vi "merFISH_resume.vi"(7 "Queue cluster":T2, 8 "Input data cluster":T1, 10 "error in":errorcluster, 11 "merFISH path":path=path "E:/") -> (1 "refnum log file":refnum<file>, 2 "Ramp":dbl[](array[numeric]), 3 "Total # z steps":i32, 4 "Ready":bool, 5 "Total # frames":i32, 6 "error out":errorcluster)   [LabVIEW 2015]
uses:
  CONTROLS/Q_PUMP_element.ctl
  CONTROLS/Q_VALVE_element.ctl
  CONTROLS/Q_DAQ_element.ctl
  CONTROLS/Q_camera_element.ctl
  CONTROLS/Q_ASI_stage_element.ctl
  CONTROLS/Q_MCL_piezo_element.ctl
  GLOBAL/Global_DAQ.vi
  GLOBAL/Global_ASI_stage.vi
  GLOBAL/Global_MCL_piezo.vi
  GLOBAL/Global_VALVE.vi
  GLOBAL/Global_PUMP.vi
  GLOBAL/Global_CAMERA.vi
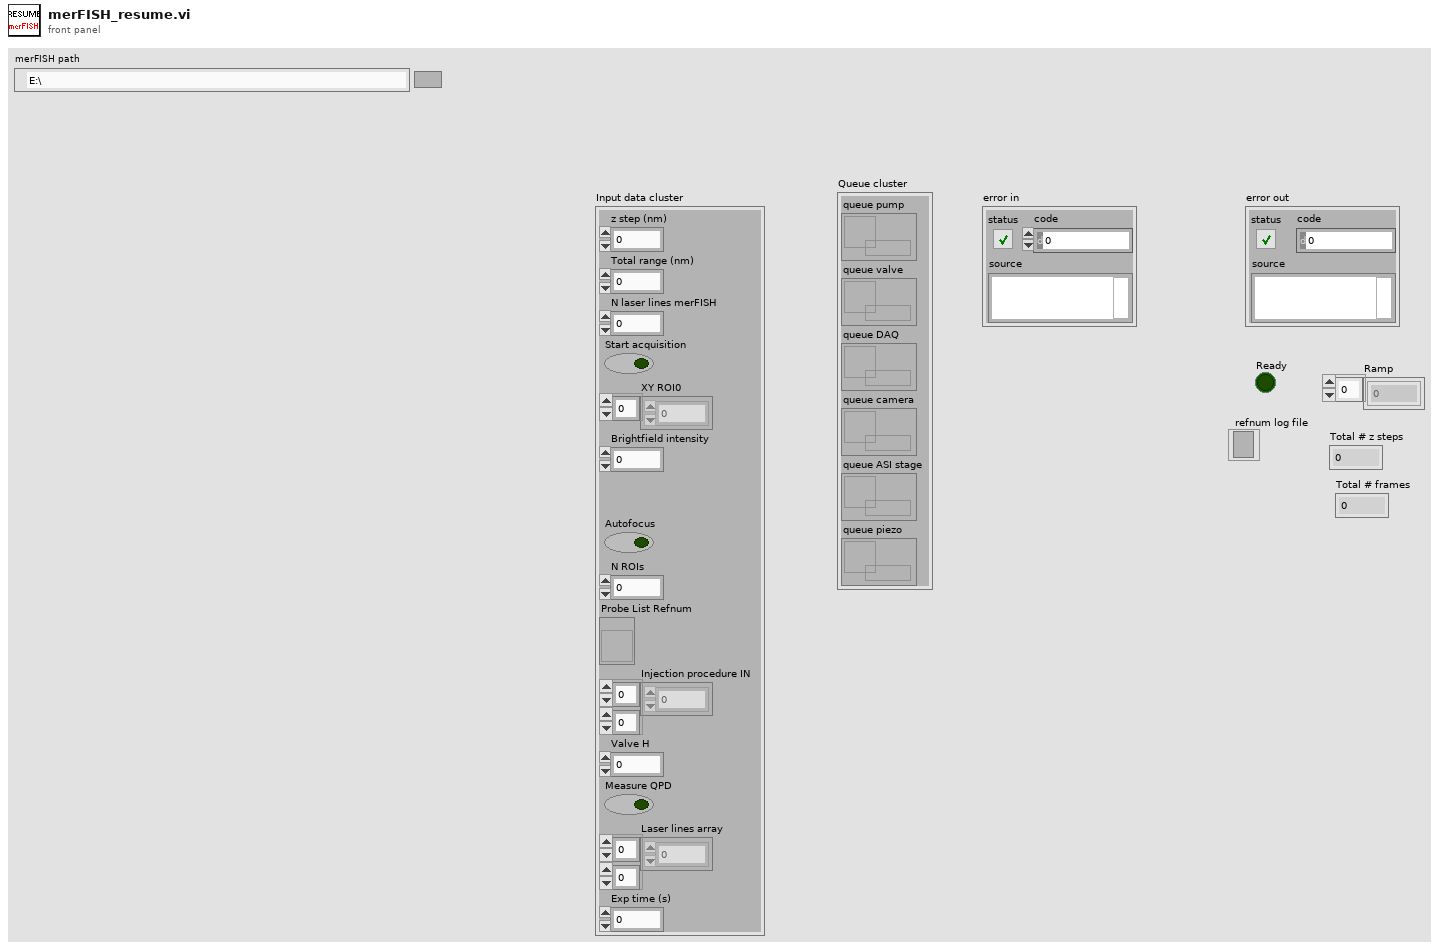
[diagram p1: front panel]
types:
  T1 = cluster{"z step (nm)":u32, "Total range (nm)":u32, "N laser lines merFISH":i32, "Start acquisition":bool, "XY ROI0":dbl[], "Brightfield intensity":dbl, "Autofocus":bool, "N ROIs":i32, "Probe List Refnum":refnum<vi>, "Injection procedure IN":i32[][], "Valve H":u8, "Measure QPD":bool, "Laser lines array":dbl[][], "Exp time (s)":sgl}
  T2 = cluster{"queue pump":refnum<queue>, "queue valve":refnum<queue>, "queue DAQ":refnum<queue>, "queue camera":refnum<queue>, "queue ASI stage":refnum<queue>, "queue piezo":refnum<queue>}
  T3 = cluster{"Laser lines array":dbl[][], "Exp time (s)":sgl}
  T4 = typedef "Q_ASI_stage_element.ctl" = cluster{"variant":variant, "Instruction":enum16{"ASI_idle", "ASI_initialize", "ASI_error", "ASI_security_stop", "ASI_read_XYZ", "ASI_up", "ASI_down", "ASI_left", "ASI_right", "ASI_save_XY", "ASI_move_to_XY", "ASI_brightfield", "ASI_init_scan", "ASI_init_merFISH", "ASI_move_to_XY_merFISH", "ASI_move_to_Z_merFISH", "ASI_init_autofocus_search_merFISH", "ASI_close_autofocus_search_merFISH", "ASI_adjust_piezo_autofocus_merFISH", "ASI_set_piezo_autofocus_to_reference_position_merFISH_TL", "ASI_close_merFISH", "ASI_stop"}}
  T5 = cluster{"XY ROI0":dbl[], "Brightfield intensity":dbl}
  T6 = typedef "Q_VALVE_element.ctl" = cluster{"variant":variant, "Instruction":enum16{"VALVE_idle", "VALVE_initialize", "VALVE_error", "VALVE_security_stop", "VALVE_change_position", "VALVE_init_merFISH", "VALVE_stop"}}
  T7 = typedef "Q_PUMP_element.ctl" = cluster{"variant":variant, "Instruction":enum16{"PUMP_idle", "PUMP_initialize", "PUMP_error", "PUMP_security_stop", "PUMP_read_pressure", "PUMP_change_pressure", "PUMP_init_merFISH", "PUMP_change_presure_merFISH", "PUMP_zero_pressure_merFISH", "PUMP_close_merFISH", "PUMP_stop"}}
  T8 = typedef "Q_DAQ_element.ctl" = cluster{"variant":variant, "Instruction":enum16{"DAQ_idle", "DAQ_initialize", "DAQ_error", "DAQ_security_stop", "DAQ_init_single_scan", "DAQ_single_scan", "DAQ_two_way_valve", "DAQ_init_merFISH", "DAQ_scan_merFISH", "DAQ_photobleaching_merFISH", "DAQ_close_merFISH", "DAQ_stop"}}
  T9 = typedef "Q_camera_element.ctl" = cluster{"variant":variant, "Instruction":enum16{"CAMERA_idle", "CAMERA_initialize", "CAMERA_error", "CAMERA_security_stop", "CAMERA_not_acquiring", "CAMERA_acquiring", "CAMERA_start_acquiring", "CAMERA_stop_acquiring", "CAMERA_change_exposure", "CAMERA_define_ROI", "CAMERA_cooler", "CAMERA_acquire_movie", "CAMERA_init_scan", "CAMERA_check_new_scan_image", "CAMERA_close_scan", "CAMERA_init_merFISH", "CAMERA_start_acquiring_merFISH", "CAMERA_close_scan_merFISH", "CAMERA_close_merFISH", "CAMERA_STOP"}}
  T10 = typedef "Q_MCL_piezo_element.ctl" = cluster{"variant":variant, "Instruction":enum16{"Piezo_idle", "Piezo_initialize", "Piezo_error", "Piezo_security_stop", "Piezo_read_z", "Piezo_move_z", "Piezo_keyboard_move", "Piezo_close_autofocus_calibration_ramp", "Piezo_change_init_state", "Piezo_init_autofocus", "Piezo_init_autofocus_merFISH_TL", "Piezo_autofocus", "Piezo_autofocus_merFISH_TL", "Piezo_stop_autofocus", "Piezo_stop_autofocus_merFISH_TL", "Piezo_autofocus_lost", "Piezo_resume_autofocus_merFISH_TL", "Piezo_check_z_position_merFISH_TL", "Piezo_init_ramp", "Piezo_move_z_ramp", "Piezo_close_ramp", "Piezo_close_merFISH", "Piezo_stop"}}
  T11 = enum16{"DAQ_idle", "DAQ_initialize", "DAQ_error", "DAQ_security_stop", "DAQ_start_QPD", "DAQ_change_QPD_display", "DAQ_read_display_QPD_signal", "DAQ_QPD_init_autofocus", "DAQ_read_display_send_QPD_signal", "DAQ_close_autofocus_calibration_ramp", "DAQ_close_autofocus", "DAQ_405", "DAQ_488", "DAQ_561", "DAQ_641", "DAQ_zero_all", "DAQ_init_single_scan", "DAQ_single_scan", "DAQ_two_way_valve", "DAQ_init_merFISH", "DAQ_scan_merFISH", "DAQ_photobleaching_merFISH", "DAQ_close_merFISH", "DAQ_init_TL", "DAQ_synchro_TL", "DAQ_close_task_TL", "DAQ_close_TL", "DAQ_stop"}
  T12 = enum16{"DAQ_idle", "DAQ_initialize", "DAQ_error", "DAQ_security_stop", "DAQ_init_single_scan", "DAQ_single_scan", "DAQ_two_way_valve", "DAQ_init_merFISH", "DAQ_scan_merFISH", "DAQ_photobleaching_merFISH", "DAQ_close_merFISH", "DAQ_stop"}
  T13 = enum16{"open", "replace", "create", "open or create", "replace or create", "replace or create with confirmation"}
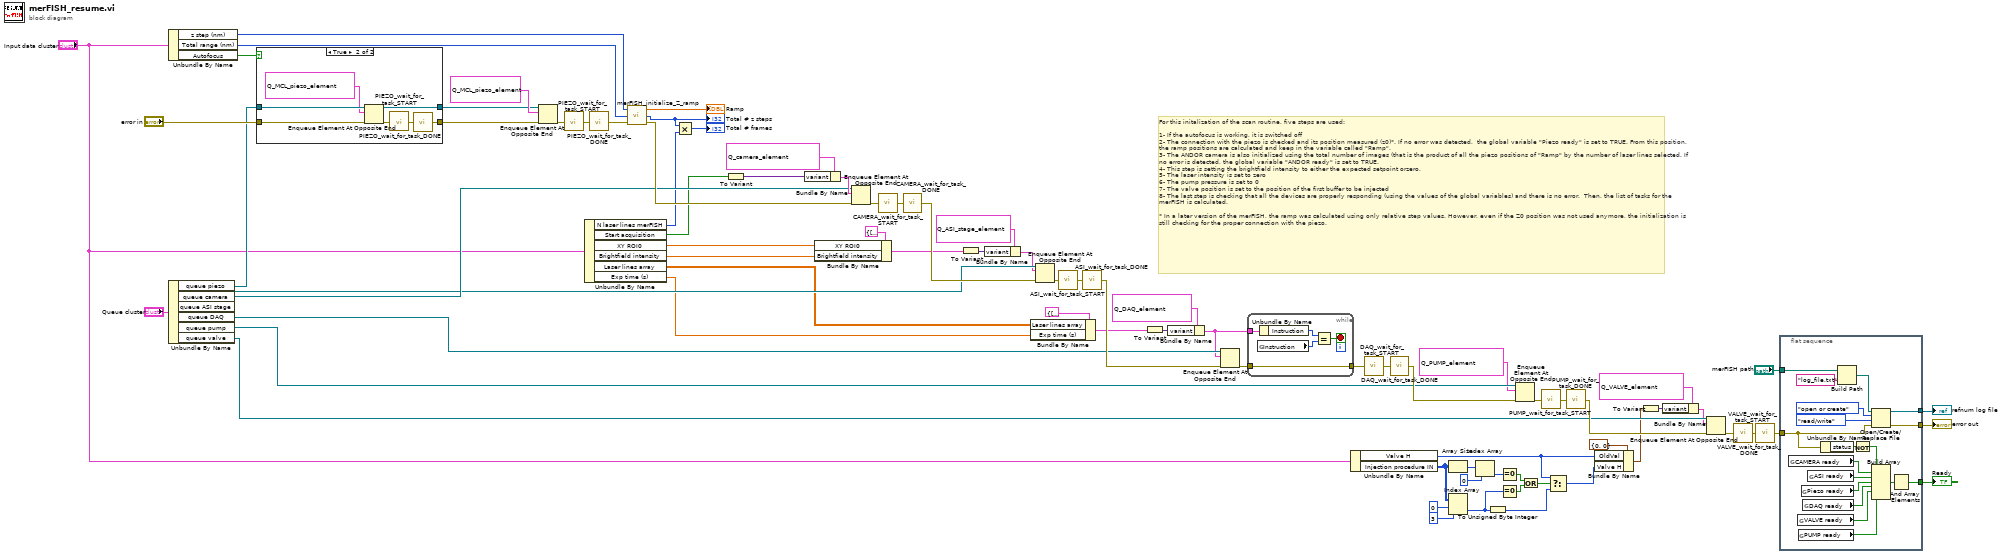
[diagram p0: block diagram]
diagram:
  # "For this initalization of the scan routine, five steps are used:\n\n1- If the autofocus is working, it is switched off\n2- The connection with the piezo is checked and its position measured (z0)*. If no error was detected,  the global variable \"Piezo ready\" is set to TRUE. From this position, the ramp positions are calculated and keep in the variable called \"Ramp\".\n3- The ANDOR camera is also initialized using the total number of images (that is the product of all the piezo positions of \"Ramp\" by the number of laser lines selected. If no error is detected, the global variable \"ANDOR ready\" is set to TRUE.\n4- This step is setting the brightfield intensity to either the expected setpoint orzero.\n5- The laser intensity is set to zero\n6- The pump pressure is set to 0\n7- The valve position is set to the position of the first buffer to be injected\n8- The last step is checking that all the devices are properly responding (using the values of the global variables) and there is no error.  Then, the list of tasks for the merFISH is calculated.\n\n* In a later version of the merFISH, the ramp was calculated using only relative step values. However, even if the Z0 position was not used anymore, the initialization is still checking for the proper connection with the piezo."
  n1 = Unbundle By Name("Input data cluster") -> ("z step (nm)"=w55:u32, "Total range (nm)"=w54:u32, "Autofocus"=w56:bool)
  n2 = Unbundle By Name("Queue cluster") -> ("queue piezo"=w60:refnum<queue>, "queue camera"=w59:refnum<queue>, "queue ASI stage"=w58:refnum<queue>, "queue DAQ"=w57:refnum<queue>, "queue pump"=w52:refnum<queue>, "queue valve"=w47:refnum<queue>)
  n3 = case shown="True" w56 {
    tunnel: w60 -> [w81 w89]
    tunnel: [w81 w88] -> w63
    tunnel: "error in" -> [w82 w86]
    tunnel: [w82 w83] -> w64
    frame False {
    }
    frame True {
      n4 = Enqueue Element At Opposite End(queue=w89, element=T10 {"variant"=variant, "Instruction"=enum."Piezo_stop_autofocus"}, error in (no error)=w86) -> (queue out=w88:refnum<queue>, error out=w85:errorcluster)  [unwired: 1 in, 1 out]
      n5 = call "PIEZO_wait_for_task_START.vi"("error in"=w85) -> ("error out"=w84:errorcluster)
      n6 = call "PIEZO_wait_for_task_DONE.vi"("error in"=w84) -> ("error out"=w83:errorcluster)
    }
  }
  n7 = Enqueue Element At Opposite End(queue=w63, element=T10 {"variant"=variant, "Instruction"=enum."Piezo_init_ramp"}, error in (no error)=w64) -> (error out=w80:errorcluster)  [unwired: 1 in, 2 out]
  n8 = call "PIEZO_wait_for_task_START.vi"("error in"=w80) -> ("error out"=w79:errorcluster)
  n9 = Unbundle By Name("Input data cluster") -> ("N laser lines merFISH"=w39:i32, "Start acquisition"=w37:bool, "XY ROI0"=w35:dbl[], "Brightfield intensity"=w34:dbl, "Laser lines array"=w12:dbl[][], "Exp time (s)"=w11:sgl)
  n10 = call "PIEZO_wait_for_task_DONE.vi"("error in"=w79) -> ("error out"=w77:errorcluster)
  n11 = call "merFISH_initialize_Z_ramp.vi"("error in"=w77, "Total range (nm)"=w54, "dZ (nm)"=w55) -> ("error out"=w72:errorcluster, "Total # steps"=w40:i32, "Ramp"=→"Ramp":dbl[])
  "Total # z steps" <- w40
  n12 = Multiply(x=w40, y=w39) -> (x*y=→"Total # frames":i32)
  n13 = To Variant(anything=w37) -> (Variant=w74:variant)
  n14 = Bundle By Name(cluster=T9 {"variant"=variant, "Instruction"=enum."CAMERA_init_merFISH"} ("Q_ANDOR_element"), "variant"=w74) -> (w73:T9)
  n15 = Bundle By Name(cluster=T5 {"XY ROI0"=[], "Brightfield intensity"=0.0} ("output cluster"), "XY ROI0"=w35, "Brightfield intensity"=w34) -> (w33:T5)
  n16 = Enqueue Element At Opposite End(queue=w59, element=w73, error in (no error)=w72) -> (error out=w71:errorcluster)  [unwired: 1 in, 2 out]
  n17 = call "CAMERA_wait_for_task_START.vi"("error in"=w71) -> ("error out"=w70:errorcluster)
  n18 = call "CAMERA_wait_for_task_DONE.vi"("error in"=w70) -> ("error out"=w69:errorcluster)
  n19 = To Variant(anything=w33) -> (Variant=w21:variant)
  n20 = Bundle By Name(cluster=T4 {"variant"=variant, "Instruction"=enum."ASI_init_merFISH"} ("Q_ASI_stage"), "variant"=w21) -> (w20:T4)
  n21 = Bundle By Name(cluster=T3 {"Laser lines array"=[], "Exp time (s)"=0.0} ("output cluster"), "Laser lines array"=w12, "Exp time (s)"=w11) -> (w13:T3)
  n22 = Enqueue Element At Opposite End(queue=w58, element=w20, error in (no error)=w69) -> (error out=w19:errorcluster)  [unwired: 1 in, 2 out]
  n23 = call "ASI_wait_for_task_START.vi"("error in"=w19) -> ("error out"=w18:errorcluster)
  n24 = call "ASI_wait_for_task_DONE.vi"("error in"=w18) -> ("error out"=w68:errorcluster)
  n25 = To Variant(anything=w13) -> (Variant=w17:variant)
  n26 = Bundle By Name(cluster=T8 {"variant"=variant, "Instruction"=enum."DAQ_init_merFISH"} ("Q_DAQ"), "variant"=w17) -> (w1:T8)
  n27 = Enqueue Element At Opposite End(queue=w57, element=w1, error in (no error)=w68) -> (error out=w3:errorcluster)  [unwired: 1 in, 2 out]
  n28 = while {
    tunnel: w3 -> [w91]
    tunnel: [w91] -> w2
    tunnel: w1 -> [w90]
    stop <- w93 stop-if-true
    n29 = global read "Global_DAQ.vi" "Instruction"() -> (w94:T11)
    n30 = Unbundle By Name(w90) -> ("Instruction"=w92:T12)
    n31 = Equal?(x=w92, y=w94) -> (x = y?=w93:bool)
  }
  n32 = Unbundle By Name("Input data cluster") -> ("Valve H"=w31:u8, "Injection procedure IN"=w30:i32[][])
  n33 = call "DAQ_wait_for_task_START.vi"("error in"=w2) -> ("error out"=w67:errorcluster)
  n34 = call "DAQ_wait_for_task_DONE.vi"("error in"=w67) -> ("error out"=w53:errorcluster)
  n35 = Array Size(array=w30) -> (size(s)=w27:i32[])
  n36 = Index Array(array=w30, index (row)=0, index (col)=3 ("disabled index (col)")) -> (element=w7:i32)
  n37 = Index Array(array=w27, index=0) -> (element=w29:i32)
  n38 = To Unsigned Byte Integer(number=w7) -> (unsigned 8bit integer=w6:u8)
  n39 = Equal To 0?(x=w29) -> (x = 0?=w10:bool)
  n40 = Equal To 0?(x=w7) -> (x = 0?=w9:bool)
  n41 = Enqueue Element At Opposite End(queue=w52, element=T7 {"variant"=variant, "Instruction"=enum."PUMP_init_merFISH"}, error in (no error)=w53) -> (error out=w50:errorcluster)  [unwired: 1 in, 2 out]
  n42 = Or(x=w10, y=w9) -> (x .or. y?=w8:bool)
  n43 = call "PUMP_wait_for_task_START.vi"("error in"=w50) -> ("error out"=w49:errorcluster)
  n44 = Select(t=w31, s=w8, f=w6) -> (s? t:f=w32:u8)
  n45 = call "PUMP_wait_for_task_DONE.vi"("error in"=w49) -> ("error out"=w48:errorcluster)
  n46 = Bundle By Name(cluster=cluster{"Valve H":u8, "OldVal":u8} {"Valve H"=0, "OldVal"=0} ("valve positions"), "OldVal"=w31, "Valve H"=w32) -> (w23:cluster{"Valve H":u8, "OldVal":u8})
  n47 = To Variant(anything=w23) -> (Variant=w45:variant)
  n48 = Bundle By Name(cluster=T6 {"variant"=variant, "Instruction"=enum."VALVE_init_merFISH"} ("element"), "variant"=w45) -> (w44:T6)
  n49 = Enqueue Element At Opposite End(queue=w47, element=w44, error in (no error)=w48) -> (error out=w43:errorcluster)  [unwired: 1 in, 2 out]
  n50 = call "VALVE_wait_for_task_START.vi"("error in"=w43) -> ("error out"=w42:errorcluster)
  n51 = call "VALVE_wait_for_task_DONE.vi"("error in"=w42) -> ("error out"=w41:errorcluster)
  n52 = flat-sequence {
    tunnel: [w112] -> w65
    tunnel: w41 -> [w98]
    tunnel: [w96] -> w66
    tunnel: "merFISH path" -> [w97]
    tunnel: [w95] -> w4
    frame #0 {
      n53 = global read "Global_CAMERA.vi" "CAMERA ready"() -> (w109:bool)
      n54 = global read "Global_VALVE.vi" "VALVE ready"() -> (w104:bool)
      n55 = global read "Global_PUMP.vi" "PUMP ready"() -> (w103:bool)
      n56 = global read "Global_MCL_piezo.vi" "Piezo ready"() -> (w110:bool)
      n57 = global read "Global_DAQ.vi" "DAQ ready"() -> (w105:bool)
      n58 = global read "Global_ASI_stage.vi" "ASI ready"() -> (w111:bool)
      n59 = Unbundle By Name(w98) -> ("status"=w107:bool)
      n60 = Build Path(base path=w97, name or relative path="log_file.txt") -> (appended path=w101:path)
      n61 = Not(x=w107) -> (.not. x?=w106:bool)
      n62 = Open/Create/Replace File(file path (use dialog)=w101, error in=w98, operation (0:open)=T13."open or create", access (0:read/write)=enum16{"read/write", "read-only", "write-only"}."read/write") -> (refnum out=w95:refnum<file>, error out=w96:errorcluster)  [unwired: 2 in, 1 out]
      n63 = Build Array(w106, w109, w111, w110, w105, w104, w103) -> (w108:bool[])
      n64 = And Array Elements(Boolean array=w108) -> (logical AND=w112:bool)
    }
  }
  "error out" <- w66
  "Ready" <- w65
  "refnum log file" <- w4
